vi "Dashboard Main.vi"() -> ()   [LabVIEW 2014]
uses:
  <vilib>/event_ctls.llb/eventvkey.ctl
  <vilib>/Rock Robotics/WPI/Dashboard/WPI_DashboardLogging Global.vi
  <vilib>/Rock Robotics/Network Tables/SD Read Boolean Array.vi
  <vilib>/Rock Robotics/Network Tables/SD Write Numeric Array.vi
  <vilib>/Rock Robotics/Network Tables/SD Write Boolean Array.vi
  <vilib>/Rock Robotics/Network Tables/SD Write Boolean.vi
  <vilib>/Rock Robotics/Network Tables/SD Read Number.vi
  <vilib>/Rock Robotics/Network Tables/SD Write String.vi
  <vilib>/Utility/config.llb/Write Key (String).vi
  <vilib>/Utility/config.llb/Write Key (I32).vi
  <vilib>/Utility/config.llb/NI_LVConfig.lvlib
panel:
  in  "Mimic <--> XBox":bool
  in  "TCP":refnum<k5>
  in  "Rec Mode":enum32{"Stop", "Record", "Playback"}(radio)
  in  "Vision":u16(ring) items=["Camera Off", "USB Camera SW", "USB Camera HW", "IP Camera"]
  out "Camera IP":string
  out "Image Message":string="Timeout in Camera Communications"
  in  "Dashboard Tab":T1(tab)
  in  "Wrist 2":bool
  in  "UA":bool
  in  "LA":bool
  in  "Camera Settings":T2={"Frame Rate"=30, "Compression"=30, "Size"=1} {"Frame Rate" scale=1.0..30.0; "Size" items=["640x480", "320x240", "160x120"]}
  out "Gyro":dbl(knob) scale=0.0..360.0
  out "JS1 Z":dbl(slide) scale=-1.0..1.0 scale format="%#_2e"
  out "JS1 Graph":cluster{"X":dbl, "Y":dbl}[](graph)
  out "JS1 Buttons":T3
  out "JS2 Z":dbl(slide) scale=-1.0..1.0 scale format="%#_2e"
  out "JS2 Graph":cluster{"X":dbl, "Y":dbl}[](graph)
  out "JS2 Buttons":T3
  out "Mode":T4(ring)=enum."Auto Disabled"
  in  "DB Camera Config":bool
  out "fps":dbl format="%#.1g"
  out "Mbps":dbl format="%#.1g"
  out "Mbps 2":bool
  in  "stop":bool
  in  "DB/String 9":string
  in  "DB/String 8":string
  in  "DB/String 7":string
  in  "DB/String 6":string
  in  "DB/String 5":string
  in  "DB/String 4":string
  in  "DB/String 3":string
  in  "DB/String 2":string
  in  "DB/String 1":string
  in  "DB/String 0":string
  in  "DB/Slider 0":dbl(slide) scale=0.0..5.0
  in  "DB/Slider 1":dbl(slide) scale=0.0..5.0
  in  "DB/Slider 2":dbl(slide) scale=0.0..5.0
  in  "DB/Slider 3":dbl(slide) scale=0.0..5.0
  out "DB/LED 3":bool
  out "DB/LED 2":bool
  out "DB/LED 1":bool
  out "DB/LED 0":bool
  in  "DB/Button 3":bool
  in  "DB/Button 2":bool
  in  "DB/Button 1":bool
  in  "DB/Button 0":bool caption="New Name"
  in  "Wrist Control\nInversion":bool
  in  "Heading Trim":dbl
  in  "Lower Arm Trim":dbl
  in  "Upper Arm Trim":dbl
  out "Robot Heading":dbl
  out "Lower Arm":dbl
  out "Upper Arm":dbl
  out "Upper Arm Mimic":dbl
  out "Lower Arm Mimic":dbl
  out "Upper Limit":bool
  out "Lower Limit":bool
  out "Lower Limit UA":bool
  out "Lower Limit LA":bool
  out "Upper Limit UA":bool
  out "Upper Limit LA":bool
  in  "stop 2":bool caption="MIMIC"
  in  "Autonomous Strategy":string(combo)
  out "Wrist":dbl
  in  "Test Slider":dbl(slide) scale=0.0..100.0 scale format="%#_3g"
  in  "On/Off":bool caption="Solenoid"
  in  "Test Name":u16(ring) items=["Select the test to run...", "Example Test", "-------------------------------", "List of tests is built in robot code.", "Replace with your own automated tests."]
  in  "Test Tree":string(tree)
  in  "Motor":cluster{"Value":dbl, "Enable":bool} {"Value" scale=-1.0..1.0 scale format="%#_3g"}
  out "Progress":T5 {"Test Progress" scale=0.0..100.0}
  in  "Rev/Fwd":cluster{"Forward":bool, "Reverse":bool}
  in  "Test Ring":u16(ring) items=["Monochrome", "Color"]
  in  "Listbox":i32(listbox)
  out "Tree":string(tree)
  out "Camera Image":T6(plugin-control)
  out "Boolean":bool
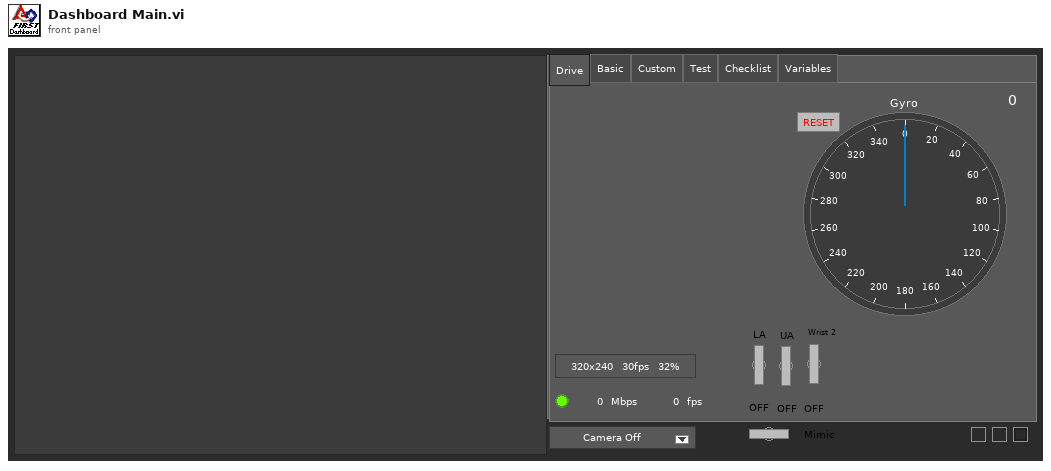
[diagram p1: front panel]
types:
  T1 = enum32{"Drive", "Basic", "Custom", "Test", "Checklist", "Variables"}
  T2 = cluster{"Frame Rate":i32, "Compression":i32, "Size":u16}
  T3 = cluster{bool, bool, bool, bool, bool, bool, bool, bool, bool, bool, bool, bool}
  T4 = enum8{"Tele-Op Disabled", "Tele-Op Enabled", "Auto Disabled", "Auto Enabled", "Test Disabled", "Test Enabled", "Disconnected", "No Code", "E-Stop"}
  T5 = cluster{"Test Progress":u8, "Test Progress Text":string}
  T6 = typedef "IMAQ Image.ctl" = refnum<image>
  T7 = typedef "Image Type" = u32
  T8 = cluster{"Camera Image":refnum<vi>, "Dashboard Tab":refnum<vi>, "Boolean":refnum<vi>, "Vision":refnum<vi>, "Rec Mode":refnum<vi>, "Test Slider":refnum<vi>, "On/Off ":refnum<vi>, "Test Ring":refnum<vi>, "Rev/Fwd":refnum<vi>, "Test Name":refnum<vi>, "Motor":refnum<vi>, "Progress":refnum<vi>, "CheckList":refnum<vi>, "Tree":refnum<vi>, "Test Tree":refnum<vi>}
  T9 = cluster{"Error Strings":string, "Disable Counts":cluster{u16, u16}, "Rail Faults":cluster{u16, u16, u16}, "Robot IP":string, "DB Mode":u8, "Event Info":cluster{"Name":string, "Type":u8, "Number":u16, "Replay":u8}, "Camera Addr":string}
  T10 = cluster{"Storage":cluster{"Disk Free":u64, "RAM Block":u32, "RAM free":u32}, "CPU Utilization":cluster{"CPU % ISR":sgl, "CPU % Time Crit":sgl, "CPU % Timed Str":sgl, "CPU % High":sgl, "CPU % Above":sgl, "CPU % Normal":sgl, "CPU % Low":sgl}, "CAN":cluster{"% Bus Utilization":sgl, "Bus Off Cnt":u32, "TX_FIFO Full Cnt":u32, "Receive Error Cnt":u8, "Transmit Error Cnt":u8}, "HID":cluster{"HID Outputs":u32, "Rumble Low":u16, "Rumble High":u16}[]}
  T11 = cluster{"Status bits":cluster{"Test Mode":bool, "Autonomous":bool, "Enabled":bool, "Code Start":bool, "Brownout":bool, "Reserved 2":bool, "Reserved 3":bool, "E-Stop":bool}, "Code Trace":cluster{"Disabled":bool, "TeleOp":bool, "Auto":bool, "Test":bool}, "Controller Type":enum16{"unknown", "cRIO", "roboRio"}, "Code?":enum16{"unknown", "noCode", "code"}, "Battery V":dbl}
  T12 = cluster{"Control Bits":cluster{"TestMode":bool, "Autonomous":bool, "Enabled":bool, "FMS Present":bool, bool, bool, bool, "E-Stop":bool}, "Team Station ":u8, "Countdown":sgl, "Joystick Values":cluster{"Axes":dbl[], "Buttons":bool[], "POVs":i16[]}[]}
  T13 = cluster{"Axes":dbl[], "Buttons":bool[], "POVs":i16[]}[]
  T14 = cluster{"Boolean Array[0]":bool, "Boolean Array[1]":bool, "Boolean Array[2]":bool, "Boolean Array[3]":bool, "Boolean Array[4]":bool, "Boolean Array[5]":bool, "Boolean Array[6]":bool, "Boolean Array[7]":bool, "Boolean Array[8]":bool}
  T15 = cluster{"Numeric Array[0]":dbl, "Numeric Array[1]":dbl, "Numeric Array[2]":dbl, "Numeric Array[3]":dbl, "Numeric Array[4]":dbl, "Numeric Array[5]":dbl, "Numeric Array[6]":dbl, "Numeric Array[7]":dbl, "Numeric Array[8]":dbl}
  T16 = cluster{"Lower Arm Trim":dbl, "Upper Arm Trim":dbl, "Heading Trim":dbl}
  T17 = cluster{"Axes":dbl[], "Buttons":bool[], "POVs":i16[]}
  T18 = cluster{"Buttons[0]":bool, "Buttons[1]":bool, "Buttons[2]":bool, "Buttons[3]":bool, "Buttons[4]":bool, "Buttons[5]":bool, "Buttons[6]":bool, "Buttons[7]":bool, "Buttons[8]":bool, "Buttons[9]":bool, "Buttons[10]":bool, "Buttons[11]":bool}
  T19 = typedef "NI_LVConfig.lvlib/Config Data RefNum.ctl" = refnum<k1>
  T20 = cluster{"Operation":enum16{"Update", "Clear"}, "Color Box":u32}[]
  T21 = typedef "eventvkey.ctl" = enum16{"ASCII", "Enter", "Return", "Shift", "Ctrl", "Alt", "Cmd", "Opt", "Caps", "NumLock", "Clear", "Break", "Up", "Down", "Left", "Right", "Insert", "Delete", "Home", "End", "PageUp", "PageDown", "Escape", "Help", "Pause", "ScrollLock", "F1", "F2", "F3", "F4", "F5", "F6", "F7", "F8", "F9", "F10", "F11", "F12", "F13", "F14", "F15", "F16", "F17", "F18", "F19", "F20", "F21", "F22", "F23", "F24", "Play", "VolumeUp", "VolumeDown", "Mute", "Two Byte Char"}
  T22 = cluster{"Image Size":bool, "Image Type":bool, "Pixel Value":bool, "ROI Information":bool, "Zoom Factor":bool}
  T23 = enum8{"Enabled", "Disabled", "Disabled and Grayed Out"}
  T24 = cluster{"Operation":enum16{"Update", "Clear"}, "Color Box":u32}
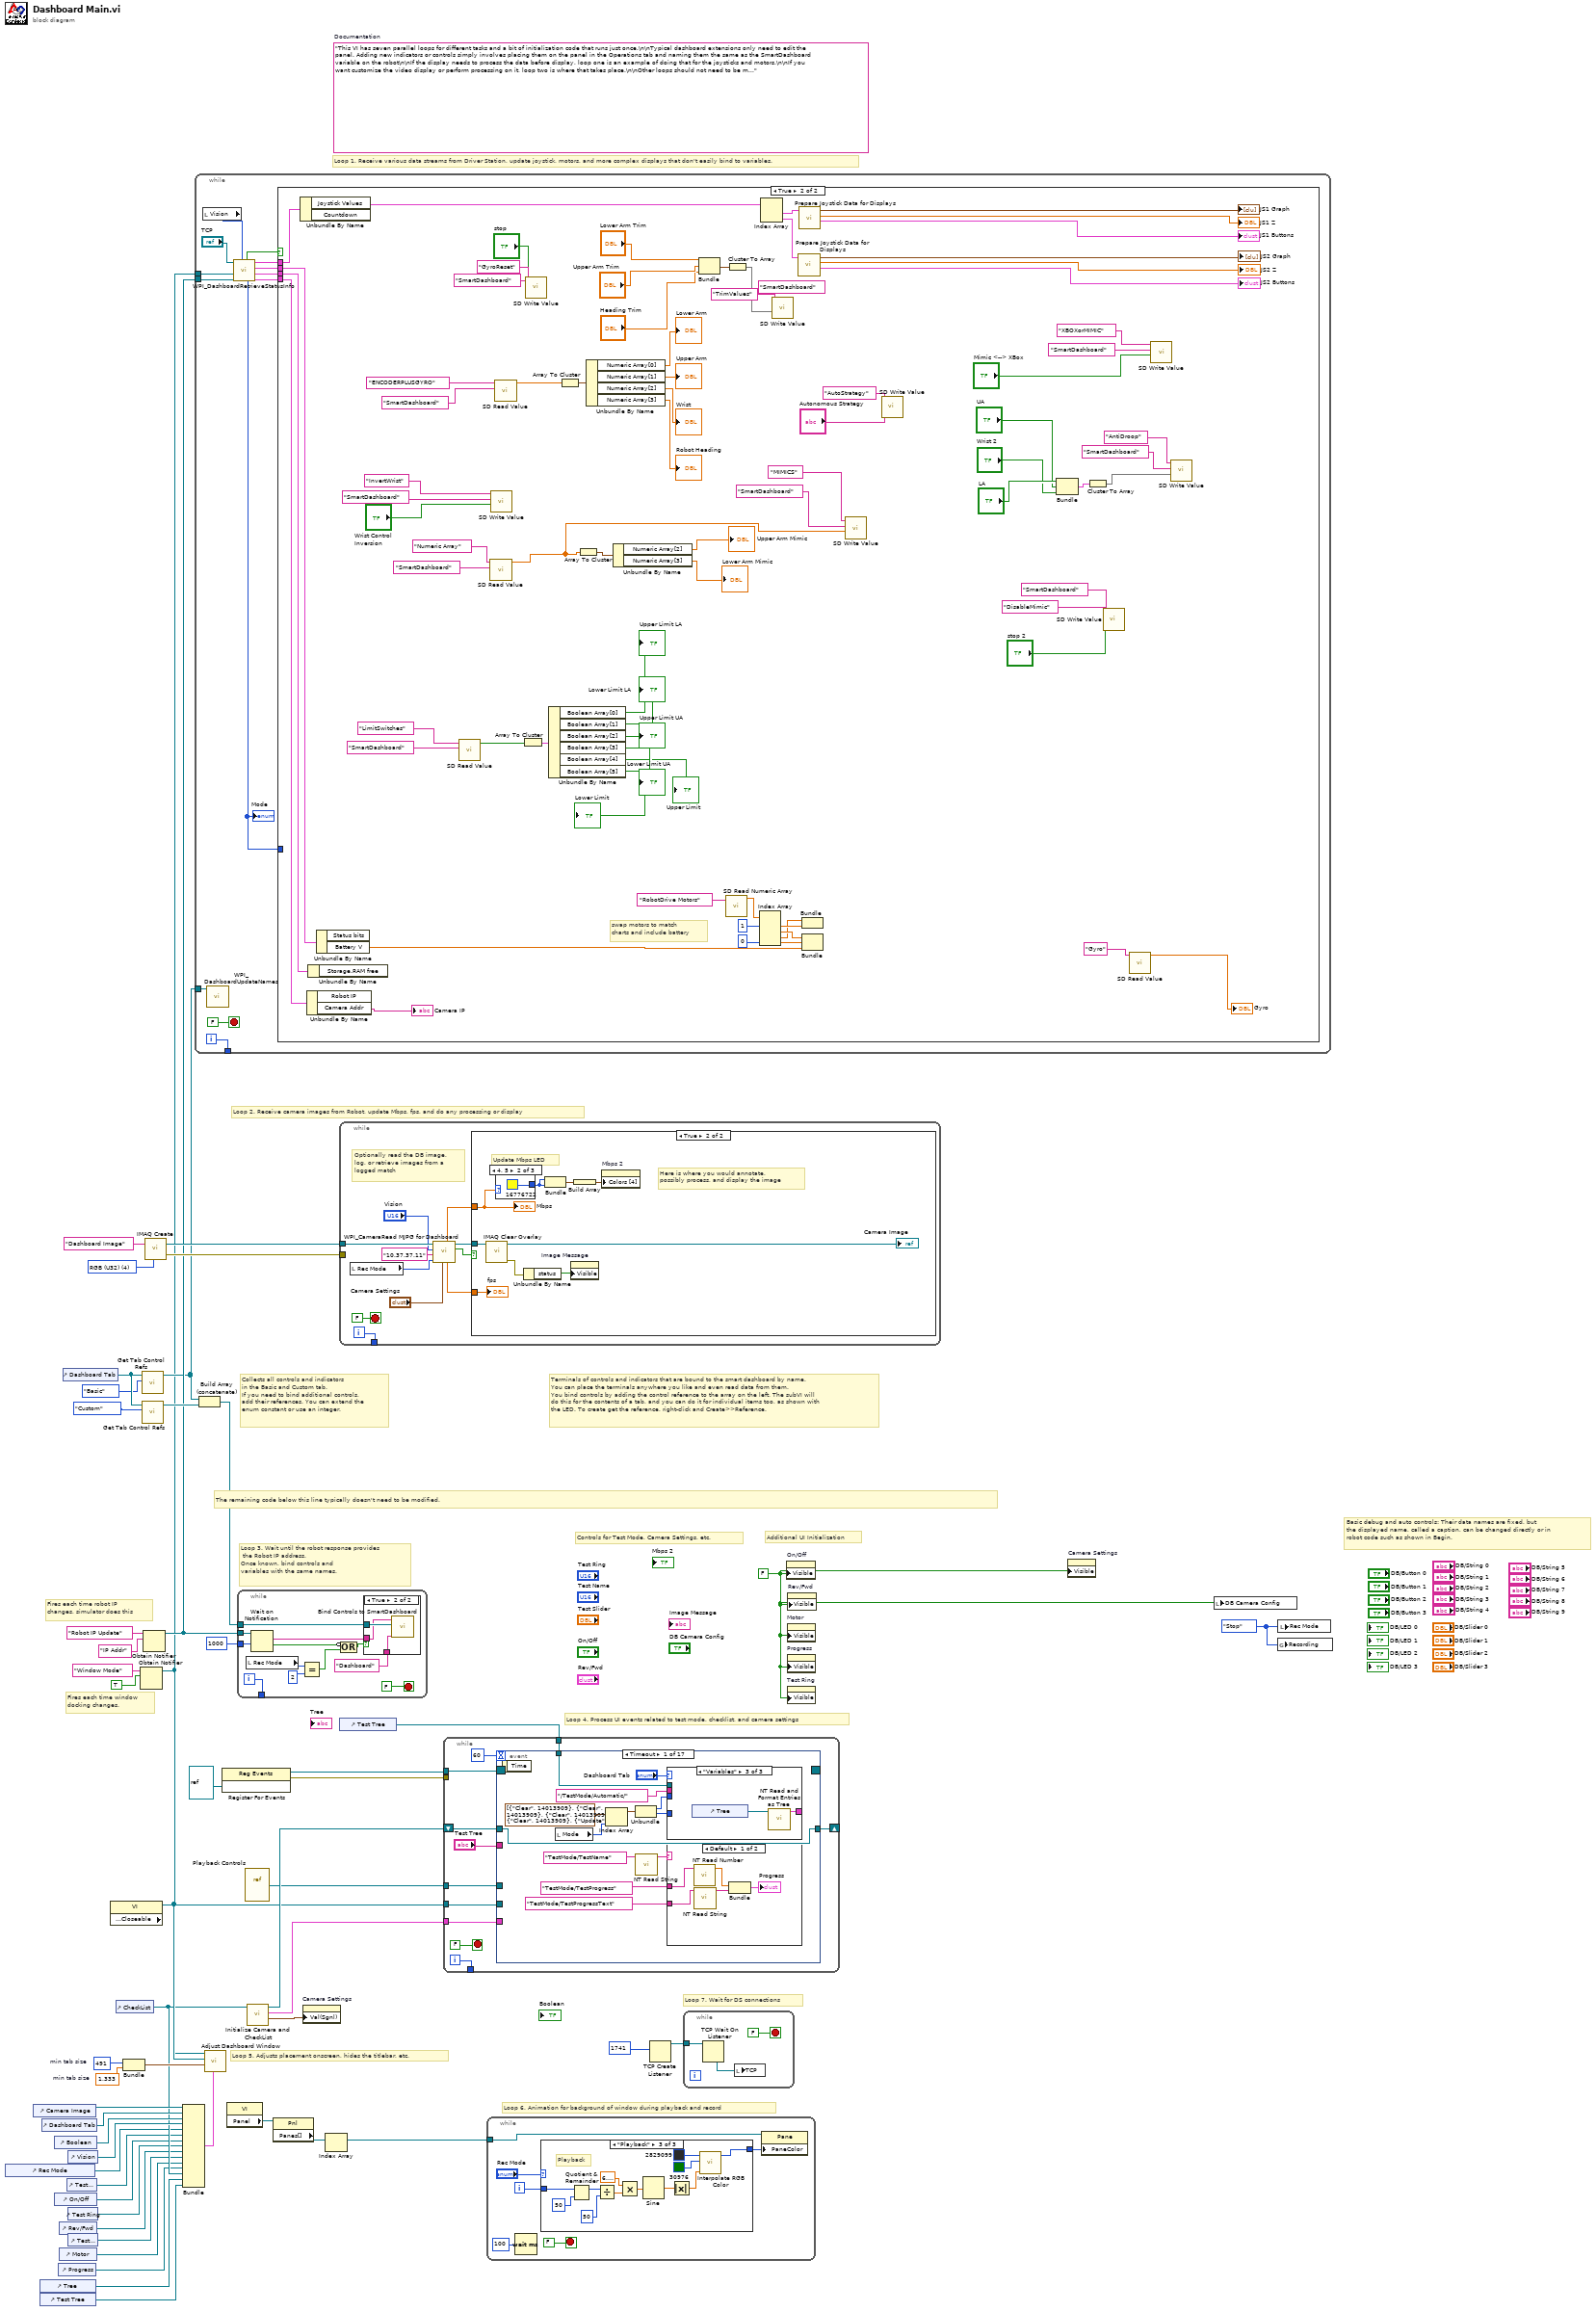
[diagram p0: block diagram]
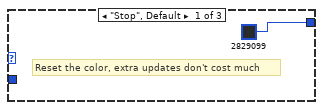
[diagram p3: hidden frame]
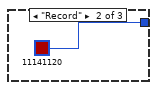
[diagram p4: hidden frame]
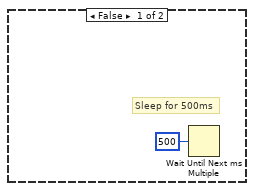
[diagram p6: hidden frame]
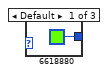
[diagram p7: hidden frame]
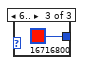
[diagram p8: hidden frame]
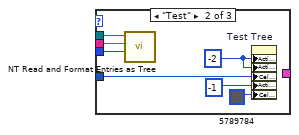
[diagram p10: hidden frame]
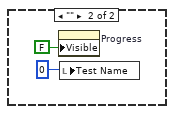
[diagram p11: hidden frame]
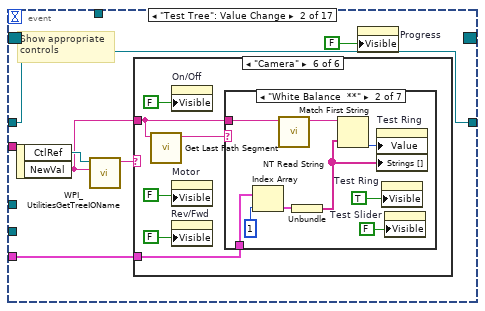
[diagram p12: hidden frame]
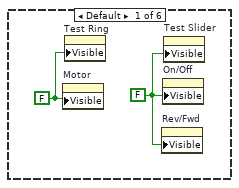
[diagram p13: hidden frame]
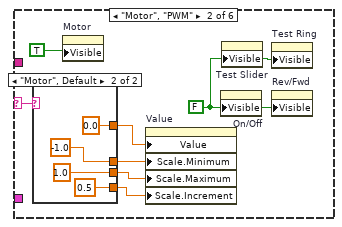
[diagram p14: hidden frame]
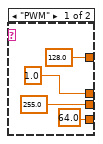
[diagram p15: hidden frame]
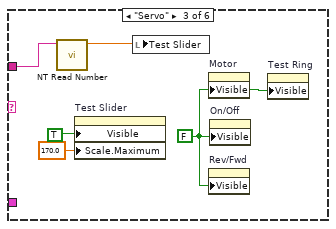
[diagram p16: hidden frame]
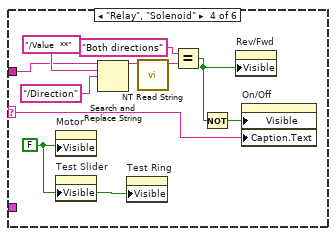
[diagram p17: hidden frame]
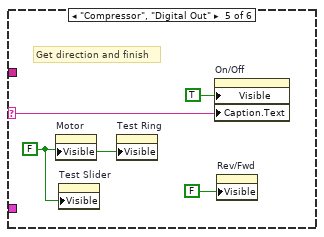
[diagram p18: hidden frame]
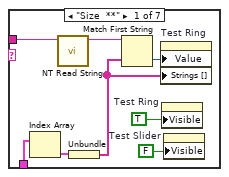
[diagram p19: hidden frame]
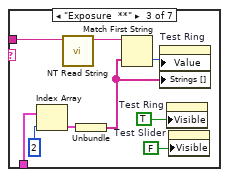
[diagram p20: hidden frame]
diagram:
  w24 = 491  # min tab size
  w23 = 1.333  # min tab size
  w32 = enum32{"Stop", "Record", "Playback"}."Stop" ("Rec Mode")
  w6 = FALSE ("Visible")
  (unwired) "This VI has seven parallel loops for different tasks and a bit of initialization code that runs just once.\n\nTypical dashboard extensions only need to edit the panel. Adding new indicators or controls simply involves placing them on the panel in the Operations tab and naming them the same as the SmartDashboard variable on the robot\n\nIf the display needs to process the data before display, loop one is an example of doing that for the joysticks and motors.\n\nIf you want customize the video display or perform processing on it, loop two is where that takes place.\n\nOther loops should not need to be modified. They are pretty standard, and document the task they perform."  # Documentation
  w52 = T7 4 items=["Grayscale (U8)", "Grayscale (I16)", "Grayscale (SGL)", "Complex (CSG)", "RGB (U32)", "HSL (U32)", "RGB (U64)"] ("Image Type")
  # "Loop 7. Wait for DS connections"
  # "Basic debug and auto controls: Their data names are fixed, but\nthe displayed name, called a caption, can be changed directly or in\nrobot code such as shown in Begin."
  # "Controls for Test Mode, Camera Settings, etc."
  # "Additional UI Initialization"
  # "Loop 6. Animation for background of window during playback and record"
  # "Fires each time robot IP\nchanges, simulator does this"
  # "Fires each time window\ndocking changes."
  # "Collects all controls and indicators\nin the Basic and Custom tab.\nIf you need to bind additional controls,\nadd their references. You can extend the\nenum constant or use an integer."
  # "The remaining code below this line typically doesn't need to be modified."
  # "Loop 4. Process UI events related to test mode, checklist, and camera settings"
  # "Terminals of controls and indicators that are bound to the smart dashboard by name.\nYou can place the terminals anywhere you like and even read data from them.\nYou bind controls by adding the control reference to the array on the left. The subVI will\ndo this for the contents of a tab, and you can do it for individual items too, as shown with\nthe LED. To create get the reference, right-click and Create>>Reference."
  # "Loop 3. Wait until the robot response provides\n the Robot IP address.\nOnce known, bind controls and\nvariables with the same names."
  # "Loop 5. Adjusts placement onscreen, hides the titlebar, etc."
  # "Loop 1. Receive various data streams from Driver Station, update joystick, motors, and more complex displays that don't easily bind to variables."
  # "Loop 2. Receive camera images from Robot, update Mbps, fps, and do any processing or display"
  n1 = control-ref of="Rec Mode"() -> (w12:refnum<vi>)
  n2 = control-ref of="Camera Image"() -> (w27:refnum<vi>)
  n3 = control-ref of="Tree"() -> (w16:refnum<vi>)
  n4 = control-ref of="Test Tree"() -> (w15:refnum<vi>)
  n5 = control-ref of="Dashboard Tab"() -> (w26:refnum<vi>)
  n6 = control-ref of="Boolean"() -> (w21:refnum<vi>)
  n7 = control-ref of="On/Off"() -> (w10:refnum<vi>)
  n8 = control-ref of="Progress"() -> (w7:refnum<vi>)
  n9 = control-ref of="Rev/Fwd"() -> (w8:refnum<vi>)
  n10 = control-ref of="Motor"() -> (w13:refnum<vi>)
  n11 = control-ref of="Dashboard Tab"() -> (w30:refnum<vi>)
  n12 = control-ref of="Test Slider"() -> (w11:refnum<vi>)
  n13 = control-ref of="Vision"() -> (w25:refnum<vi>)
  n14 = control-ref of="Test Ring"() -> (w9:refnum<vi>)
  n15 = control-ref of="Test Name"() -> (w14:refnum<vi>)
  n16 = property class="VI" props=["Front Panel.Closeable"]() -> (reference out=w31:refnum<vi>)  [unwired: 2 in, 2 out]
  n17 = control-ref of="CheckList"() -> (w17:refnum<vi>)
  n18 = Bundle("min tab size"=w24, "min tab size"=w23) -> (w22:cluster{"min tab size":i32, "min tab size":dbl})  [unwired: 1 in]
  n19 = Obtain Notifier(name (unnamed)="Window Mode", notification data type=TRUE) -> (notifier out=w3:refnum<notifier>)  [unwired: 2 in, 2 out]
  n20 = call <vilib>:"Get Tab Control Refs.vi"("Page Index"=T1."Basic" ("Dashboard Tab"), "TabControl in"=w30) -> ("ControlsOnPage"=w4:refnum<vi>[])  [unwired: 9 in]
  n21 = call <vilib>:"Get Tab Control Refs.vi"("Page Index"=T1."Custom" ("Dashboard Tab"), "TabControl in"=w30) -> ("ControlsOnPage"=w29:refnum<vi>[])  [unwired: 9 in]
  n22 = Obtain Notifier(name (unnamed)="Robot IP Update", notification data type="IP Addr" ("name (unnamed)")) -> (notifier out=w5:refnum<notifier>)  [unwired: 2 in, 2 out]
  n23 = call "IMAQ Create"("Image Name"="Dashboard Image", "Image Type"=w52) -> ("New Image"=w50:T6, "error out"=w49:errorcluster)  [unwired: 2 in, 1 out]
  n24 = Bundle("Camera Image"=w27, "Dashboard Tab"=w26, "Boolean"=w21, "Vision"=w25, "Rec Mode"=w12, "Test Slider"=w11, "On/Off"=w10, "Test Ring"=w9, "Rev/Fwd"=w8, "Test Name"=w14, "Motor"=w13, "Progress"=w7, "CheckList"=w17, "Tree"=w16, "Test Tree"=w15) -> (w18:T8)  [unwired: 1 in]
  n25 = while {
    tunnel: [w64] -> _
    tunnel: w5 -> [w58]
    tunnel: w4 -> [w57]
    tunnel: w3 -> [w53]
    i -> [w64]
    stop <- FALSE stop-if-true
    n26 = local read "Vision"() -> (w55:u16)
    n27 = call <vilib>:"WPI_DashboardUpdateNames.vi"("Controls on Tab"=w57) -> ()  [unwired: 11 in]
    n28 = call <vilib>:"WPI_DashboardRetrieveStatusInfo.vi"("Vision"=w55, "Binding Refnum"=w58, "Window Mode Notifier"=w53, "TCP Cnx"="TCP") -> ("Power and Errors"=w59:T9, "Robot Metrics"=w62:T10, "Status Info"=w63:T11, "Control Info"=w60:T12, "Robot Mode"=w56:T4, "Process?"=w61:bool)  [unwired: 2 in]
    "Mode" <- w56
    n29 = case shown="True" w61 {
      tunnel: w63 -> [_ w144]
      tunnel: w62 -> [_ w143]
      tunnel: w60 -> [_ w142]
      tunnel: w59 -> [_ w141]
      tunnel: w56 -> [_ _]
      frame False {
      }
      frame True {
        # "swap motors to match\ncharts and include battery"
        n30 = Unbundle By Name(w142) -> ("Joystick Values"=w131:T13)  [unwired: 1 out]
        n31 = Unbundle By Name(w141) -> ("Camera Addr"=→"Camera IP":string)  [unwired: 1 out]
        n32 = Unbundle By Name(w143) -> ()  [unwired: 1 out]
        n33 = Unbundle By Name(w144) -> ("Battery V"=w132:dbl)  [unwired: 1 out]
        n34 = call-poly <vilib>:"SD Read Value.vi"("Table Prefix"="SmartDashboard", "Name"="LimitSwitches") -> ("Boolean Array"=w111:bool[])  [unwired: 7 in, 2 out]
        n35 = call-poly <vilib>:"SD Read Value.vi"("Table Prefix"="SmartDashboard", "Name"="Numeric Array") -> ("Numeric Array"=w74:dbl[])  [unwired: 7 in, 2 out]
        n36 = call-poly <vilib>:"SD Write Value.vi"("Boolean"="Wrist Control\nInversion", "Table Prefix"="SmartDashboard", "Name"="InvertWrist") -> ()  [unwired: 7 in, 2 out]
        n37 = call-poly <vilib>:"SD Read Value.vi"("Table Prefix"="SmartDashboard", "Name"="ENCODERPLUSGYRO") -> ("Numeric Array"=w119:dbl[])  [unwired: 7 in, 2 out]
        n38 = Array To Cluster(array=w111) -> (cluster=w110:T14)
        n39 = call-poly <vilib>:"SD Write Value.vi"("Boolean"="stop", "Table Prefix"="SmartDashboard", "Name"="GyroReset") -> ()  [unwired: 7 in, 2 out]
        n40 = Unbundle By Name(w110) -> ("Boolean Array[0]"=→"Upper Limit LA":bool, "Boolean Array[1]"=→"Lower Limit LA":bool, "Boolean Array[2]"=→"Upper Limit UA":bool, "Boolean Array[3]"=→"Lower Limit UA":bool, "Boolean Array[4]"=→"Upper Limit":bool, "Boolean Array[5]"=→"Lower Limit":bool)
        n41 = Array To Cluster(array=w119) -> (cluster=w118:T15)
        n42 = Array To Cluster(array=w74) -> (cluster=w101:T15)
        n43 = Unbundle By Name(w118) -> ("Numeric Array[0]"=→"Lower Arm":dbl, "Numeric Array[1]"=→"Upper Arm":dbl, "Numeric Array[2]"=→"Wrist":dbl, "Numeric Array[3]"=→"Robot Heading":dbl)
        n44 = Unbundle By Name(w101) -> ("Numeric Array[2]"=→"Upper Arm Mimic":dbl, "Numeric Array[3]"=→"Lower Arm Mimic":dbl)
        n45 = Bundle("Lower Arm Trim"="Lower Arm Trim", "Upper Arm Trim"="Upper Arm Trim", "Heading Trim"="Heading Trim") -> (w78:T16)  [unwired: 1 in]
        n46 = call <vilib>:"SD Read Numeric Array.vi"("Name"="RobotDrive Motors") -> ("Numeric Array"=w134:dbl[])  [unwired: 8 in, 2 out]
        n47 = Cluster To Array(cluster=w78) -> (array=w77:dbl[])
        n48 = Index Array(array=w134, index #1=1, index #4=0) -> (element #1=w136:dbl, element #2=w137:dbl, element #3=w135:dbl, element #4=w140:dbl)  [unwired: 2 in]
        n49 = Index Array(array=w131) -> (element #1=w130:T17, element #2=w126:T17)  [unwired: 2 in]
        n50 = call-poly <vilib>:"SD Write Value.vi"("Numeric Array"=w77, "Table Prefix"="SmartDashboard", "Name"="TrimValues") -> ()  [unwired: 7 in, 2 out]
        n51 = call "Prepare Joystick Data for Displays.vi"("Joystick Values"=w126) -> ("Buttons"=→"JS2 Buttons":T18, "Z Axis"=→"JS2 Z":dbl, "Cartesian Data"=→"JS2 Graph":cluster{"X axis":dbl, "X axis":dbl}[])  [unwired: 8 in]
        n52 = call "Prepare Joystick Data for Displays.vi"("Joystick Values"=w130) -> ("Buttons"=→"JS1 Buttons":T18, "Z Axis"=→"JS1 Z":dbl, "Cartesian Data"=→"JS1 Graph":cluster{"X axis":dbl, "X axis":dbl}[])  [unwired: 8 in]
        n53 = Bundle("Numeric"=w135, "Numeric"=w136) -> ()  [unwired: 1 in, 1 out]
        n54 = Bundle("Numeric"=w137, "Numeric"=w140, "Battery V"=w132) -> ()  [unwired: 1 in, 1 out]
        n55 = call-poly <vilib>:"SD Write Value.vi"("Numeric Array"=w74, "Table Prefix"="SmartDashboard", "Name"="MIMICS") -> ()  [unwired: 7 in, 2 out]
        n56 = call-poly <vilib>:"SD Write Value.vi"("String"="Autonomous Strategy", "Name"="AutoStrategy") -> ()  [unwired: 8 in, 2 out]
        n57 = Bundle("LA"="LA", "UA"="UA", "Wrist 2"="Wrist 2") -> (w94:cluster{"LA":bool, "UA":bool, "Wrist 2":bool})  [unwired: 1 in]
        n58 = Cluster To Array(cluster=w94) -> (array=w93:bool[])
        n59 = call-poly <vilib>:"SD Write Value.vi"("Boolean"="stop 2", "Table Prefix"="SmartDashboard", "Name"="DisableMimic") -> ()  [unwired: 7 in, 2 out]
        n60 = call-poly <vilib>:"SD Read Value.vi"("Name"="Gyro") -> ("Numeric"=→"Gyro":dbl)  [unwired: 8 in, 2 out]
        n61 = call-poly <vilib>:"SD Write Value.vi"("Boolean"="Mimic <--> XBox", "Table Prefix"="SmartDashboard", "Name"="XBOXorMIMIC") -> ()  [unwired: 7 in, 2 out]
        n62 = call-poly <vilib>:"SD Write Value.vi"("Boolean Array"=w93, "Table Prefix"="SmartDashboard", "Name"="AntiDroop") -> ()  [unwired: 7 in, 2 out]
      }
    }
  }
  n63 = Build Array (concatenate)(w4, w29) -> (w28:refnum<vi>[])
  n64 = call "Adjust Dashboard Window.vi"("Sizing Refnums"=w18, "Size Constraints"=w22, "VI"=w31, "Notifier in"=w3) -> ()  [unwired: 8 in]
  n65 = register-events(refnum<vi> refnum) -> (reference out=w36:refnum<event-registration>, error out=w35:errorcluster)  [unwired: 2 in]
  n66 = property class="VI"() -> ("Panel"=w39:refnum<vi>)  [unwired: 2 in, 2 out]
  n67 = while {
    tunnel: w28 -> [w156]
    tunnel: w5 -> [w154]
    tunnel: [w152] -> _
    tunnel: u32 1000 ("milliseconds to wait") -> [w151]
    i -> [w152]
    stop <- FALSE stop-if-true
    n68 = local read "Rec Mode"() -> (w147:enum32{"Stop", "Record", "Playback"})
    n69 = Wait on Notification(notifier=w154, timeout in ms (-1)=w151) -> (notification=w153:string, timed out?=w149:bool)  [unwired: 2 in, 2 out]
    n70 = Equal?(x=w147, y=u16 2 ("Rec Mode")) -> (x = y?=w148:bool)
    n71 = Compound Arithmetic op=OR(invert w149, w148) -> (w150:bool)
    n72 = case shown="True" w150 {
      tunnel: w156 -> [_ w159]
      tunnel: w153 -> [_ w158]
      tunnel: "Dashboard" -> [_ w157]
      frame False {
      }
      frame True {
        n73 = call <vilib>:"Bind Controls to SmartDashboard.vi"("Client Name"=w157, "Bound Control Refs"=w159, "Server IP Address"=w158) -> ()  [unwired: 9 in]
      }
    }
  }
  n74 = vi-ref "Playback Controls.vi"() -> (w37:refnum<vi>)
  n75 = call "Initialize Camera and CheckList.vi"("ListBox in"=w17) -> ("Cluster"=w43:cluster{"value":i32, "value":i32, "index":i32}, "Array"=w44:cluster{string[]}[], "File Refnum"=w42:T19)  [unwired: 8 in]
  n76 = property class="Pnl"(reference=w39) -> ("Panes[]"=w40:refnum<vi>[])  [unwired: 1 in, 2 out]
  n77 = property on="Camera Settings" class="Clust (strict)"("Val(Sgnl)"=w43) -> ()  [unwired: 2 in, 2 out]
  n78 = Index Array(array=w40) -> (element=w38:refnum<vi>)  [unwired: 1 in]
  n79 = while {
    tunnel: w50 -> [w168]
    tunnel: w49 -> [_]
    tunnel: [w169] -> _
    i -> [w169]
    stop <- FALSE stop-if-true
    # "Optionally read the DB image,\nlog, or retrieve images from a\nlogged match"
    n80 = local read "Rec Mode"() -> (w162:enum32{"Stop", "Record", "Playback"})
    n81 = call <vilib>:"WPI_CameraRead MJPG for Dashboard.vi"("Camera Settings"="Camera Settings", "Rec Mode"=w162, "Camera IP"="10.37.37.11", "Camera Mode"="Vision", "Refnum in"=w168) -> ("Active"=w166:bool, "Refnum out"=w167:T6, "FPS"=w165:dbl, "Bandwidth (Mbps)"=w164:dbl)  [unwired: 3 in]
    n82 = case shown="True" w166 {
      tunnel: w167 -> [_ w175]
      tunnel: w164 -> [_ w174]
      tunnel: w165 -> [_ w172]
      frame False {
        # "Sleep for 500ms"
        n83 = Wait Until Next ms Multiple(millisecond multiple=u32 500) -> ()  [unwired: 1 out]
      }
      frame True {
        # "Here is where you would annotate,\npossibly process, and display the image"
        # "Update Mbps LED"
        n84 = call "IMAQ Clear Overlay"("Image"=w175) -> ("error out"=w179:errorcluster, "Image Out"=→"Camera Image":T6)  [unwired: 2 in, 7 out]
        n85 = case shown="4, 5" w174 {
          tunnel: [u32 6618880 ("Color Box") u32 16776722 ("Color Box") u32 16716800 ("Color Box")] -> w176
          frame Default {
          }
          frame 4, 5 {
          }
          frame 6.. {
          }
        }
        n86 = Unbundle By Name(w179) -> ("status"=w180:bool)
        n87 = Bundle("Color Box"=w176, "Color Box"=w176) -> (w178:cluster{"Color Box":u32, "Color Box":u32})  [unwired: 1 out]
        n88 = property on="Image Message" class="Str"("Visible"=w180) -> ()  [unwired: 2 in, 2 out]
        n89 = Build Array(w178) -> (w177:cluster{"Color Box":u32, "Color Box":u32}[])
        n90 = property on="Mbps 2" class="Bool (strict)"("Colors [4]"=w177) -> ()  [unwired: 2 in, 2 out]
        "Mbps" <- w174
        "fps" <- w172
      }
    }
  }
  n91 = control-ref of="Test Tree"() -> (w41:refnum<vi>)
  n92 = while {
    tunnel: w44 -> [w191]
    shift-right: [w190] -> _
    shift-left: w42 -> [w189]
    tunnel: [w188] -> _
    tunnel: w41 -> [w187]
    tunnel: w37 -> [w186]
    tunnel: w36 -> [w185]
    tunnel: w35 -> [_]
    tunnel: w31 -> [w184]
    i -> [w188]
    stop <- FALSE stop-if-true
    n93 = event shown="[0] Timeout" {
      selector: w185 -> [_ _ _ _ _ _ _ _ _ _ _ _ _ _ _ _ _]
      dyn-events: [_ _ _ _ _ _ _ _ _ _ _ _ _ w429 _ _ _] -> _
      timeout: u32 60 ("milliseconds to wait") -> [_ _ _ _ _ _ _ _ _ _ _ _ _ _ _ _ _]
      tunnel: w187 -> [w203 _ _ _ _ _ _ _ _ _ _ _ _ _ _ _ _]
      tunnel: "Test Tree" -> [_ _ _ _ _ _ _ _ w398 w406 w408 w412 w420 _ _ _ _]
      tunnel: w191 -> [_ w225 _ _ _ _ w362 w392 _ _ _ _ _ _ _ _ _]
      tunnel: [w199 w224 w323 w328 w336 w348 w361 w385 w397 w404 w407 w411 w419 w431 w445 w446 w456] -> w190
      tunnel: w189 -> [w199 w224 w323 w328 w336 w348 w360 w385 w397 w404 w407 w411 w419 w431 w445 w446 w456]
      tunnel: w186 -> [_ _ _ _ _ _ _ _ _ _ _ _ _ w432 _ w449 _]
      tunnel: w184 -> [_ _ _ _ _ _ _ _ _ _ _ _ _ w427 _ _ _]
      event Timeout {
        n94 = event-data() -> ()  [unwired: 1 in, 1 out]
        n95 = local read "Mode"() -> (w202:T4)
        n96 = Index Array(array=T20 [{"Operation"=enum."Clear", "Color Box"=14013909}, {"Operation"=enum."Clear", "Color Box"=14013909}, {"Operation"=enum."Clear", "Color Box"=14013909}, {"Operation"=enum."Clear", "Color Box"=14013909}, {"Operation"=enum."Update", "Color Box"=14013909}, {"Operation"=enum."Update", "Color Box"=16777215}, {"Operation"=enum."Clear", "Color Box"=14013909}, {"Operation"=enum."Clear", "Color Box"=14013909}, {"Operation"=enum."Clear", "Color Box"=14013909}], index=w202) -> (element=w197:T24)
        n97 = Unbundle(w197) -> ("Operation"=w196:enum16{"Update", "Clear"}, "Color Box"=w195:u32)
        n98 = call <vilib>:"NT Read String.vi"("Name"="TestMode/TestName") -> ("String"=w206:string)  [unwired: 9 in, 1 out]
        n99 = case shown="\"Variables\"" "Dashboard Tab" {
          tunnel: w203 -> [_ w214 _]
          tunnel: "/TestMode/Automatic/" ("Name Pattern") -> [_ w213 _]
          tunnel: w196 -> [_ w212 _]
          tunnel: [_ _ w216] -> _
          tunnel: w195 -> [_ w208 _]
          frame "Custom", Default {
          }
          frame "Test" {
            w211 = -2 ("Active Item:Row Number")
            n100 = call <vilib>:"NT Read and Format Entries as Tree.vi"("Operation"=w212, "Name Pattern"=w213, "Tree Refnum"=w214) -> ()  [unwired: 7 in, 2 out]
            n101 = property on="Test Tree" class="Tree (strict)"("Active Item Row Number"=w211, "ActiveColNum"=w211, "CellBG"=w208, "Active Item Row Number"=-1 ("Active Item:Row Number"), "CellBG"=u32 5789784 ("Color Box")) -> ()  [unwired: 2 in, 2 out]
          }
          frame "Variables" {
            n102 = control-ref of="Tree"() -> (w215:refnum<vi>)
            n103 = call <vilib>:"NT Read and Format Entries as Tree.vi"("Tree Refnum"=w215) -> ("Formatted Strings"=w216:cluster{"Name":string, "Value":string}[])  [unwired: 9 in, 1 out]
          }
        }
        n104 = case shown="Default" w206 {
          tunnel: "TestMode/TestProgress" ("Name") -> [w218 _]
          tunnel: "TestMode/TestProgressText" ("Name") -> [w217 _]
          frame Default {
            n105 = call <vilib>:"NT Read Number.vi"("Name"=w218) -> ("Numeric"=w219:dbl)  [unwired: 9 in, 1 out]
            n106 = call <vilib>:"NT Read String.vi"("Name"=w217) -> ("String"=w220:string)  [unwired: 9 in, 1 out]
            n107 = Bundle("Numeric"=w219, "String"=w220) -> (→"Progress":cluster{"Numeric":dbl, "String":string})  [unwired: 1 in]
          }
          frame "" {
            n108 = property on="Progress" class="Clust (strict)"("Visible"=FALSE) -> ()  [unwired: 2 in, 2 out]
            n109 = local write "Test Name"(u16 0) -> ()
          }
        }
      }
      event "Test Tree": Value Change {
        # "Show appropriate\ncontrols"
        n110 = event-data() -> ("CtlRef"=w228:refnum<vi>, "NewVal"=w226:string)  [unwired: 1 in]
        n111 = call <vilib>:"WPI_UtilitiesGetTreeIOName.vi"("NewVal"=w226, "TreeControl in"=w228) -> ("I/O Name"=w229:string)  [unwired: 9 in]
        n112 = case shown="\"Camera\"" w229 {
          selector: w229 -> [_ w236 _ w254 w263 _]
          tunnel: w226 -> [_ _ w251 w253 _ w270]
          tunnel: w225 -> [_ _ _ _ _ w269]
          frame Default {
            w231 = FALSE ("Visible")
            w230 = FALSE ("Visible")
            n113 = property on="Motor" class="Clust (strict)"("Visible"=w230) -> ()  [unwired: 2 in, 2 out]
            n114 = property on="Test Ring" class="Ring (strict)"("Visible"=w230) -> ()  [unwired: 2 in, 2 out]
            n115 = property on="Rev/Fwd" class="Clust (strict)"("Visible"=w231) -> ()  [unwired: 2 in, 2 out]
            n116 = property on="On/Off" class="Bool (strict)"("Visible"=w231) -> ()  [unwired: 2 in, 2 out]
            n117 = property on="Test Slider" class="Slide (strict)"("Visible"=w231) -> ()  [unwired: 2 in, 2 out]
          }
          frame "Motor", "PWM" {
            w237 = FALSE ("Visible")
            n118 = case shown="\"Motor\", Default" w236 {
              tunnel: [1.0 ("Value") -1.0 ("Value")] -> w235
              tunnel: [255.0 ("Value") 1.0 ("Value")] -> w234
              tunnel: [128.0 ("Value") 0.0 ("Value")] -> w233
              tunnel: [64.0 ("Value") 0.5 ("Value")] -> w232
              frame "PWM" {
              }
              frame "Motor", Default {
              }
            }
            n119 = property on="Motor" class="Clust (strict)"("Visible"=TRUE) -> ()  [unwired: 2 in, 2 out]
            n120 = property on="Value" class="Slide (strict)"("Value"=w233, "Scale.Minimum"=w235, "Scale.Maximum"=w234, "Scale.Increment"=w232) -> ()  [unwired: 2 in, 2 out]
            n121 = property on="On/Off" class="Bool (strict)"("Visible"=w237) -> ()  [unwired: 2 in, 2 out]
            n122 = property on="Test Slider" class="Slide (strict)"("Visible"=w237) -> ()  [unwired: 2 in, 2 out]
            n123 = property on="Test Ring" class="Ring (strict)"("Visible"=w237) -> ()  [unwired: 2 in, 2 out]
            n124 = property on="Rev/Fwd" class="Clust (strict)"("Visible"=w237) -> ()  [unwired: 2 in, 2 out]
          }
          frame "Servo" {
            w249 = FALSE ("Visible")
            n125 = call <vilib>:"NT Read Number.vi"("Name"=w251) -> ("Numeric"=w250:dbl)  [unwired: 9 in, 1 out]
            n126 = property on="Test Slider" class="Slide (strict)"("Visible"=TRUE, "Scale.Maximum"=170.0 ("Scale.Range:Maximum")) -> ()  [unwired: 2 in, 2 out]
            n127 = local write "Test Slider"(w250) -> ()
            n128 = property on="Motor" class="Clust (strict)"("Visible"=w249) -> ()  [unwired: 2 in, 2 out]
            n129 = property on="Rev/Fwd" class="Clust (strict)"("Visible"=w249) -> ()  [unwired: 2 in, 2 out]
            n130 = property on="On/Off" class="Bool (strict)"("Visible"=w249) -> ()  [unwired: 2 in, 2 out]
            n131 = property on="Test Ring" class="Ring (strict)"("Visible"=w249) -> ()  [unwired: 2 in, 2 out]
          }
          frame "Relay", "Solenoid" {
            w252 = FALSE ("Visible")
            n132 = property on="Motor" class="Clust (strict)"("Visible"=w252) -> ()  [unwired: 2 in, 2 out]
            n133 = property on="Test Slider" class="Slide (strict)"("Visible"=w252) -> ()  [unwired: 2 in, 2 out]
            n134 = Search and Replace String(input string=w253, search string="/Value  **", replace string="/Direction") -> (result string=w259:string)  [unwired: 5 in, 3 out]
            n135 = property on="Test Ring" class="Ring (strict)"("Visible"=w252) -> ()  [unwired: 2 in, 2 out]
            n136 = call <vilib>:"NT Read String.vi"("Name"=w259) -> ("String"=w257:string)  [unwired: 9 in, 1 out]
            n137 = Equal?(x="Both directions", y=w257) -> (x = y?=w255:bool)
            n138 = Not(x=w255) -> (.not. x?=w256:bool)
            n139 = property on="Rev/Fwd" class="Clust (strict)"("Visible"=w255) -> ()  [unwired: 2 in, 2 out]
            n140 = property on="On/Off" class="Bool (strict)"("Visible"=w256, "Caption.Text"=w254) -> ()  [unwired: 2 in, 2 out]
          }
          frame "Compressor", "Digital Out" {
            w262 = FALSE ("Visible")
            # "Get direction and finish"
            n141 = property on="Motor" class="Clust (strict)"("Visible"=w262) -> ()  [unwired: 2 in, 2 out]
            n142 = property on="Test Slider" class="Slide (strict)"("Visible"=w262) -> ()  [unwired: 2 in, 2 out]
            n143 = property on="Test Ring" class="Ring (strict)"("Visible"=w262) -> ()  [unwired: 2 in, 2 out]
            n144 = property on="On/Off" class="Bool (strict)"("Visible"=TRUE, "Caption.Text"=w263) -> ()  [unwired: 2 in, 2 out]
            n145 = property on="Rev/Fwd" class="Clust (strict)"("Visible"=FALSE) -> ()  [unwired: 2 in, 2 out]
          }
          frame "Camera" {
            n146 = call <vilib>:"Get Last Path Segment.vi"("String in"=w270) -> ("String out"=w271:string)  [unwired: 10 in]
            n147 = property on="On/Off" class="Bool (strict)"("Visible"=FALSE) -> ()  [unwired: 2 in, 2 out]
            n148 = property on="Motor" class="Clust (strict)"("Visible"=FALSE) -> ()  [unwired: 2 in, 2 out]
            n149 = property on="Rev/Fwd" class="Clust (strict)"("Visible"=FALSE) -> ()  [unwired: 2 in, 2 out]
            n150 = case shown="\"White Balance  **\"" w271 {
              tunnel: w270 -> [w277 w286 w295 w304 w313 _ w319]
              tunnel: w269 -> [w275 w283 w292 w301 w310 _ _]
              frame "Size  **" {
                n151 = Index Array(array=w275) -> (element=w274:cluster{string[]})  [unwired: 1 in]
                n152 = call <vilib>:"NT Read String.vi"("Name"=w277) -> ("String"=w276:string)  [unwired: 9 in, 1 out]
                n153 = Unbundle(w274) -> (w272:string[])
                n154 = Match First String(2:w272, 3:w276) -> (0:w273:i32)  [unwired: 1 out]
                n155 = property on="Test Ring" class="Ring (strict)"("Value"=w273, "Strings []"=w272) -> ()  [unwired: 2 in, 2 out]
                n156 = property on="Test Ring" class="Ring (strict)"("Visible"=TRUE) -> ()  [unwired: 2 in, 2 out]
                n157 = property on="Test Slider" class="Slide (strict)"("Visible"=FALSE) -> ()  [unwired: 2 in, 2 out]
              }
              frame "White Balance  **" {
                n158 = Index Array(array=w283, index=1) -> (element=w284:cluster{string[]})
                n159 = call <vilib>:"NT Read String.vi"("Name"=w286) -> ("String"=w285:string)  [unwired: 9 in, 1 out]
                n160 = Unbundle(w284) -> (w281:string[])
                n161 = Match First String(2:w281, 3:w285) -> (0:w280:i32)  [unwired: 1 out]
                n162 = property on="Test Ring" class="Ring (strict)"("Value"=w280, "Strings []"=w281) -> ()  [unwired: 2 in, 2 out]
                n163 = property on="Test Ring" class="Ring (strict)"("Visible"=TRUE) -> ()  [unwired: 2 in, 2 out]
                n164 = property on="Test Slider" class="Slide (strict)"("Visible"=FALSE) -> ()  [unwired: 2 in, 2 out]
              }
              frame "Exposure  **" {
                n165 = Index Array(array=w292, index=2) -> (element=w293:cluster{string[]})
                n166 = call <vilib>:"NT Read String.vi"("Name"=w295) -> ("String"=w294:string)  [unwired: 9 in, 1 out]
                n167 = Unbundle(w293) -> (w289:string[])
                n168 = Match First String(2:w289, 3:w294) -> (0:w290:i32)  [unwired: 1 out]
                n169 = property on="Test Ring" class="Ring (strict)"("Value"=w290, "Strings []"=w289) -> ()  [unwired: 2 in, 2 out]
                n170 = property on="Test Ring" class="Ring (strict)"("Visible"=TRUE) -> ()  [unwired: 2 in, 2 out]
                n171 = property on="Test Slider" class="Slide (strict)"("Visible"=FALSE) -> ()  [unwired: 2 in, 2 out]
              }
              frame "Exposure Priority  **" {
                n172 = Index Array(array=w301, index=3) -> (element=w302:cluster{string[]})
                n173 = call <vilib>:"NT Read String.vi"("Name"=w304) -> ("String"=w303:string)  [unwired: 9 in, 1 out]
                n174 = Unbundle(w302) -> (w298:string[])
                n175 = Match First String(2:w298, 3:w303) -> (0:w299:i32)  [unwired: 1 out]
                n176 = property on="Test Ring" class="Ring (strict)"("Value"=w299, "Strings []"=w298) -> ()  [unwired: 2 in, 2 out]
                n177 = property on="Test Ring" class="Ring (strict)"("Visible"=TRUE) -> ()  [unwired: 2 in, 2 out]
                n178 = property on="Test Slider" class="Slide (strict)"("Visible"=FALSE) -> ()  [unwired: 2 in, 2 out]
              }
              frame "Color Enable  **" {
                n179 = Index Array(array=w310, index=4) -> (element=w311:cluster{string[]})
                n180 = call <vilib>:"NT Read String.vi"("Name"=w313) -> ("String"=w312:string)  [unwired: 9 in, 1 out]
                n181 = Unbundle(w311) -> (w307:string[])
                n182 = Match First String(2:w307, 3:w312) -> (0:w308:i32)  [unwired: 1 out]
                n183 = property on="Test Ring" class="Ring (strict)"("Value"=w308, "Strings []"=w307) -> ()  [unwired: 2 in, 2 out]
                n184 = property on="Test Ring" class="Ring (strict)"("Visible"=TRUE) -> ()  [unwired: 2 in, 2 out]
                n185 = property on="Test Slider" class="Slide (strict)"("Visible"=FALSE) -> ()  [unwired: 2 in, 2 out]
              }
              frame Default {
                n186 = property on="Test Ring" class="Ring (strict)"("Visible"=FALSE) -> ()  [unwired: 2 in, 2 out]
                n187 = property on="Test Slider" class="Slide (strict)"("Visible"=FALSE) -> ()  [unwired: 2 in, 2 out]
              }
              frame "Brightness  **", "Color Level  **", "Compression  **", "FPS  **", "Sharpness  **" {
                n188 = call <vilib>:"NT Read Number.vi"("Name"=w319) -> ("Numeric"=w318:dbl)  [unwired: 9 in, 1 out]
                n189 = local write "Test Slider"(w318) -> ()
                n190 = property on="Test Slider" class="Slide (strict)"("Visible"=TRUE, "Scale.Maximum"=100.0 ("Scale.Range:Maximum")) -> ()  [unwired: 2 in, 2 out]
                n191 = property on="Test Ring" class="Ring (strict)"("Visible"=FALSE) -> ()  [unwired: 2 in, 2 out]
              }
            }
          }
        }
        n192 = property on="Progress" class="Clust (strict)"("Visible"=FALSE) -> ()  [unwired: 2 in, 2 out]
      }
      event "Test Name": Mouse Enter {
        # "Populate the ring with the list of tests"
        n193 = event-data() -> ()  [unwired: 1 in, 1 out]
        n194 = call <vilib>:"NT Read String Array.vi"("Name"="TestMode/TestList") -> ("String Array"=w327:string[])  [unwired: 9 in, 1 out]
        n195 = Build Array (concatenate)("Select the test to run...", w327) -> (w326:string[])
        n196 = property on="Test Name" class="Ring (strict)"("Strings []"=w326) -> ()  [unwired: 2 in, 2 out]
      }
      event "Test Name": Value Change {
        w329 = FALSE ("Visible")
        # "Tell the robot the test name to run"
        n197 = event-data() -> ("NewVal"=w333:u16)  [unwired: 1 in]
        n198 = property on="Test Name" class="Ring (strict)"() -> ("Strings []"=w334:string[])  [unwired: 2 in, 2 out]
        n199 = local write "Progress"(T5 {"Test Progress"=0, "Test Progress Text"=""} ("Progress")) -> ()
        n200 = Index Array(array=w334, index=w333) -> (element=w332:string)
        n201 = call <vilib>:"NT Write String.vi"("String"=w332, "Name"="TestMode/TestName") -> ()  [unwired: 9 in, 1 out]
        n202 = property on="Progress" class="Clust (strict)"("Visible"=TRUE) -> ()  [unwired: 2 in, 2 out]
        n203 = property on="Motor" class="Clust (strict)"("Visible"=w329) -> ()  [unwired: 2 in, 2 out]
        n204 = property on="Test Slider" class="Slide (strict)"("Visible"=w329) -> ()  [unwired: 2 in, 2 out]
        n205 = property on="On/Off" class="Bool (strict)"("Visible"=w329) -> ()  [unwired: 2 in, 2 out]
        n206 = property on="Rev/Fwd" class="Clust (strict)"("Visible"=w329) -> ()  [unwired: 2 in, 2 out]
        n207 = property on="Test Ring" class="Ring (strict)"("Visible"=w329) -> ()  [unwired: 2 in, 2 out]
      }
      event "Listbox": Double Click {
        # "Shift clears all"
        # "Update symbols on the listbox"
        n208 = event-data() -> ("PlatMods.Shift"=w337:bool, "Row"=w339:i32)  [unwired: 1 in]
        n209 = case shown="True" w337 {
          tunnel: w339 -> [w343 _]
          tunnel: 1 -> [w342 _]
          frame False {
            n210 = property on="Listbox" class="LstBox (strict)"() -> ("Item Symbols"=w341:i32[])  [unwired: 2 in, 2 out]
            n211 = Replace Array Subset(array=w341, new element=w342, index=w343) -> (w340:i32[])
            n212 = property on="Listbox" class="LstBox (strict)"("Item Symbols"=w340) -> ()  [unwired: 2 in, 2 out]
          }
          frame True {
            w344 = 0 ("Top Row")
            n213 = property on="Listbox" class="LstBox (strict)"() -> ("Number of Rows"=w346:u32)  [unwired: 2 in, 2 out]
            n214 = Initialize Array(0, w346) -> (w345:i32[])
            n215 = property on="Listbox" class="LstBox (strict)"("Top Row"=w344, "Value"=w344, "Item Symbols"=w345) -> ()  [unwired: 2 in, 2 out]
          }
        }
      }
      event "Listbox": Key Down {
        # "Update symbols on the listbox\nLeft and right keys check and uncheck"
        n216 = event-data() -> ("VKey"=w350:T21)  [unwired: 1 in]
        n217 = case shown="\"Left\", \"Right\"" w350 {
          selector: w350 -> [w355 _]
          tunnel: eventvkey."Left" ("VKey") -> [w353 _]
          frame "Left", "Right" {
            n218 = Equal?(x=w353, y=w355) -> (x = y?=w354:bool)
            n219 = Select(t=0, s=w354, f=1) -> (s? t:f=w356:i32)
            n220 = property on="Listbox" class="LstBox (strict)"() -> ("Item Symbols"=w359:i32[])  [unwired: 2 in, 2 out]
            n221 = Replace Array Subset(array=w359, new element=w356, index="Listbox") -> (w358:i32[])
            n222 = property on="Listbox" class="LstBox (strict)"("Item Symbols"=w358) -> ()  [unwired: 2 in, 2 out]
          }
          frame Default {
          }
        }
      }
      event "DB Camera Config": Value Change {
        # "Show or hide the cluster of controls, store in ini file"
        n223 = event-data() -> ("NewVal"=w363:bool)  [unwired: 1 in]
        n224 = case shown="False" w363 {
          tunnel: w362 -> [w372 _]
          tunnel: [w365 w383] -> w361
          tunnel: w360 -> [w364 w383]
          frame False {
            w379 = "Camera"
            w382 = FALSE ("Visible")
            n225 = local read "Camera Settings"() -> (w371:T2)
            n226 = Index Array(array=w372) -> (element=w375:cluster{string[]})  [unwired: 1 in]
            n227 = Unbundle(w371) -> ("Frame Rate"=w370:i32, "Compression"=w369:i32, "Size"=w373:u16)
            n228 = Unbundle(w375) -> (w374:string[])
            n229 = Index Array(array=w374, index=w373) -> (element=w368:string)
            n230 = call-poly <vilib>:"Write Key.vi"("section"=w379, "value"=w368, "key"="Size", "refnum"=w364) -> ("refnum out"=w381:T19)  [unwired: 2 in, 5 out]
            n231 = call-poly <vilib>:"Write Key.vi"("section"=w379, "value"=w370, "key"="FrameRate", "refnum"=w381) -> ("refnum out"=w380:T19)  [unwired: 1 in, 6 out]
            n232 = property on="Camera Settings" class="Clust (strict)"("Visible"=w382) -> ()  [unwired: 2 in, 2 out]
            n233 = local write "DB Camera Config"(w382) -> ()
            n234 = call-poly <vilib>:"Write Key.vi"("section"=w379, "value"=w369, "key"="Compression", "refnum"=w380) -> ("refnum out"=w366:T19)  [unwired: 1 in, 6 out]
            n235 = call <vilib>:"Close Config Data.vi"("refnum"=w366) -> ("file path"=w367:path)  [unwired: 2 in, 8 out]
            n236 = call <vilib>:"Open Config Data.vi"("configuration file path"=w367) -> ("refnum"=w365:T19)  [unwired: 8 in, 2 out]
          }
          frame True {
            n237 = property on="Camera Settings" class="Clust (strict)"("Visible"=TRUE) -> ()  [unwired: 2 in, 2 out]
          }
        }
      }
      event "Camera Settings": Value Change {
        # "Update summary string when any elements of DB camera change"
        n238 = event-data() -> ("NewVal"=w396:T2)  [unwired: 1 in]
        n239 = Index Array(array=w392) -> (element=w391:cluster{string[]})  [unwired: 1 in]
        n240 = Unbundle(w396) -> ("Frame Rate"=w387:i32, "Compression"=w386:i32, "Size"=w389:u16)
        n241 = Unbundle(w391) -> (w390:string[])
        n242 = Index Array(array=w390, index=w389) -> (element=w388:string)
        n243 = Format Into String(format string="%s   %dfps   %d%%", w388, w387, w386) -> (resulting string=w393:string)  [unwired: 2 in, 1 out]
        n244 = Build Array(w393) -> (w394:string[])
        n245 = property on="DB Camera Config" class="Bool (strict)"("Strings [4]"=w394) -> ()  [unwired: 2 in, 2 out]
      }
      event "Motor.Enable": Value Change {
        # "When the test mode otor enable helper is set, update that\ntree row item's value"
        n246 = event-data() -> ("NewVal"=w402:bool)  [unwired: 1 in]
        n247 = Unbundle("Motor") -> ("Value"=w401:dbl)  [unwired: 1 out]
        n248 = Select(t=w401, s=w402, f=0.0) -> (s? t:f=w399:dbl)
        n249 = call <vilib>:"NT Write Number.vi"("Numeric"=w399, "Name"=w398) -> ()  [unwired: 9 in, 1 out]
      }
      event "Test Slider": Value Change {
        # "When the test mode slider helper is set, update that\ntree row item's value"
        n250 = event-data() -> ("NewVal"=w405:dbl)  [unwired: 1 in]
        n251 = call <vilib>:"NT Write Number.vi"("Numeric"=w405, "Name"=w406) -> ()  [unwired: 9 in, 1 out]
      }
      event "On/Off": Value Change {
        # "When the test mode on/off helper value is set, update that\ntree row item's value"
        n252 = event-data() -> ("NewVal"=w410:bool)  [unwired: 1 in]
        n253 = Boolean To (0,1)(Boolean=w410) -> (0, 1=w409:i16)
        n254 = call <vilib>:"NT Write Number.vi"("Numeric"=w409, "Name"=w408) -> ()  [unwired: 9 in, 1 out]
      }
      event "Rev/Fwd": Value Change {
        # "When the test mode helper value for relays is set, update that\ntree row item's value"
        n255 = event-data() -> ("NewVal.Forward"=w418:bool, "NewVal.Reverse"=w417:bool)  [unwired: 1 in]
        n256 = Boolean To (0,1)(Boolean=w418) -> (0, 1=w414:i16)
        n257 = Boolean To (0,1)(Boolean=w417) -> (0, 1=w416:i16)
        n258 = Negate(x=w416) -> (-x=w415:i16)
        n259 = Add(x=w414, y=w415) -> (x+y=w413:i16)
        n260 = call <vilib>:"NT Write Number.vi"("Numeric"=w413, "Name"=w412) -> ()  [unwired: 9 in, 1 out]
      }
      event "Test Ring": Value Change {
        # "When a test mode helper value is selected from the ring,\nset the tree item's variable to the string value"
        n261 = event-data() -> ("NewVal"=w422:u16)  [unwired: 1 in]
        n262 = property on="Test Ring" class="Ring (strict)"() -> ("Strings []"=w423:string[])  [unwired: 2 in, 2 out]
        n263 = Index Array(array=w423, index=w422) -> (element=w421:string)
        n264 = call <vilib>:"NT Write String.vi"("String"=w421, "Name"=w420) -> ()  [unwired: 9 in, 1 out]
      }
      event "Rec Mode": Value Change {
        # "Update globals for recording mode and path to read log from.\nClear when logging and let NetworkTables set path for vision to\nuse."
        n265 = event-data() -> ("NewVal"=w433:enum32{"Stop", "Record", "Playback"})  [unwired: 1 in]
        n266 = global write "WPI_DashboardLogging Global.vi" "Logging Filename"(path "") -> ()
        n267 = case shown="\"Playback\"" w433 {
          tunnel: w432 -> [_ w435 w443]
          tunnel: [_ _ w442] -> w429
          tunnel: [_ _ w441] -> _
          tunnel: w427 -> [_ _ w439]
          tunnel: cluster{i32, i32} {-250, 170} -> [_ _ w438]
          tunnel: [_ _ T22 {"Image Size"=TRUE, "Image Type"=TRUE, "Pixel Value"=TRUE, "ROI Information"=TRUE, "Zoom Factor"=FALSE} ("Image Information Shown:All Elements")] -> w425
          tunnel: [_ _ TRUE ("Zoom Factor")] -> w424
          frame Default {
          }
          frame "Stop", "Record" {
            # "Place Window too"
            n268 = invoke class="VI" method="FP.Close"(reference=w435) -> (reference out=w434:refnum<vi>)  [unwired: 2 in, 2 out]
            n269 = invoke class="VI" method="Abort VI"(reference=w434) -> ()  [unwired: 2 in, 3 out]
          }
          frame "Playback" {
            n270 = call "Open Playback Panel.vi"("Offset"=w438, "DB VI Ref"=w439, "Playback in"=w443) -> ("Playback out"=w440:refnum<vi>)  [unwired: 8 in]
            n271 = register-events(w440) -> (reference out=w442:refnum<event-registration>, error out=w441:errorcluster)  [unwired: 2 in]
          }
        }
        n272 = global write "WPI_DashboardLogging Global.vi" "Recording"(w433) -> ()
        n273 = property on="Camera Image" class="ImageControl"("Image Information Shown"=w425, "Image Information Visible"=w424) -> ()  [unwired: 2 in, 2 out]
        n274 = call <vilib>:"WPI_DashboardNT Log FieldName Cache.vi"("Operation"=enum16{"Lookup/Add", "Index", "Clear"}."Clear") -> ()  [unwired: 8 in, 3 out]
      }
      event Panel Close {
        w444 = enum32{"Stop", "Record", "Playback"}."Stop" ("Rec Mode")
        # "Playback window has been closed, abort"
        n275 = event-data() -> ()  [unwired: 1 in, 4 out]
        n276 = local write "Rec Mode"(w444) -> ()
        n277 = global write "WPI_DashboardLogging Global.vi" "Recording"(w444) -> ()
      }
      event Panel Close {
        # "Abort playback window and ourself"
        n278 = event-data() -> ()  [unwired: 1 in, 4 out]
        n279 = invoke class="VI" method="FP.Close"(reference=w449) -> (reference out=w448:refnum<vi>)  [unwired: 2 in, 2 out]
        n280 = invoke class="VI" method="Abort VI"(reference=w448) -> (error out=w447:errorcluster)  [unwired: 2 in, 2 out]
        n281 = invoke class="VI" method="Abort VI"(error in=w447) -> ()  [unwired: 2 in, 3 out]
      }
      event "Vision": Value Change {
        # "Enable/Disable Compression slider.\nHW USB is hard-coded into the camera"
        n282 = event-data() -> ("NewVal"=w455:u16)  [unwired: 1 in]
        n283 = Equal?(x=w455, y=u32 2 ("milliseconds to wait")) -> (x = y?=w453:bool)
        n284 = Select(t=T23."Disabled and Grayed Out" ("Disabled"), s=w453, f=T23."Enabled" ("Disabled")) -> (s? t:f=w450:T23)
        n285 = property on="Compression" class="Slide (strict)"("DisabledEnum"=w450) -> ()  [unwired: 2 in, 2 out]
      }
    }
  }
  n286 = while {
    tunnel: w38 -> [w458]
    i -> [w461]
    stop <- FALSE stop-if-true
    n287 = Wait (ms)(milliseconds to wait=u32 100) -> ()  [unwired: 1 out]
    n288 = case shown="\"Playback\"" "Rec Mode" {
      tunnel: w461 -> [_ _ w476]
      tunnel: [u32 2829099 ("Base Color") u32 11141120 ("Target Color") w465] -> w457
      frame "Stop", Default {
        # "Reset the color, extra updates don't cost much"
      }
      frame "Record" {
      }
      frame "Playback" {
        # "Playback"
        n289 = Quotient & Remainder(x=w476, y=u32 50 ("milliseconds to wait")) -> (x-y*floor(x/y)=w472:u32)  [unwired: 1 out]
        n290 = Divide(x=w472, y=u32 50 ("milliseconds to wait")) -> (x/y=w469:dbl)
        n291 = Multiply(x=6.283185307179586, y=w469) -> (x*y=w474:dbl)
        n292 = Sine(x=w474) -> (sin(x)=w473:dbl)
        n293 = Absolute Value(x=w473) -> (abs(x)=w466:dbl)
        n294 = call "Interpolate RGB Color.vi"("Proportion"=w466, "Target Color"=u32 30976, "Base Color"=u32 2829099) -> ("Result Color"=w465:u32)  [unwired: 8 in]
      }
    }
    n295 = property class="Pane"(reference=w458, "PaneColor"=w457) -> ()  [unwired: 1 in, 2 out]
  }
  n296 = TCP Create Listener(10:u16 1741 ("timeout ms (25000)")) -> (3:w1:refnum<k5>)  [unwired: 4 in, 2 out]
  n297 = while {
    tunnel: w1 -> [w478]
    stop <- FALSE stop-if-true
    n298 = TCP Wait On Listener(11:w478) -> (4:w477:refnum<k5>)  [unwired: 3 in, 4 out]
    n299 = local write "TCP"(w477) -> ()
  }
  n300 = property on="On/Off" class="Bool (strict)"("Visible"=w6) -> ()  [unwired: 2 in, 2 out]
  n301 = property on="Motor" class="Clust (strict)"("Visible"=w6) -> ()  [unwired: 2 in, 2 out]
  n302 = property on="Progress" class="Clust (strict)"("Visible"=w6) -> ()  [unwired: 2 in, 2 out]
  n303 = property on="Test Ring" class="Ring (strict)"("Visible"=w6) -> ()  [unwired: 2 in, 2 out]
  n304 = property on="Rev/Fwd" class="Clust (strict)"("Visible"=w6) -> ()  [unwired: 2 in, 2 out]
  n305 = property on="Camera Settings" class="Clust (strict)"("Visible"=w6) -> ()  [unwired: 2 in, 2 out]
  n306 = local write "DB Camera Config"(w6) -> ()
  n307 = global write "WPI_DashboardLogging Global.vi" "Recording"(w32) -> ()
  n308 = local write "Rec Mode"(w32) -> ()
